vi "PQfetchTables.vi"(8 "error in":errorcluster, 10 "res":u32, 11 "conn":u32) -> (0 "error out":errorcluster, 1 "Data":string[](array[string]), 2 "res_out":u32, 3 "conn_out":u32, 4 "PQnTuples":i32, 6 "PQnFields":i32)   [LabVIEW 2019, in "libpqutility.lvlib"]
doc: "Fetch Result Data from DatabaseRequest into String Array.\nSee PostgreSQL c-lib doku for further information."
uses:
  libpqutility.lvlib
  libpqlv/libpqlv.lvlib
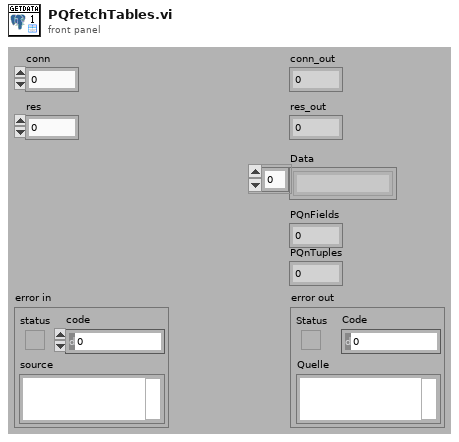
[diagram p1: front panel]
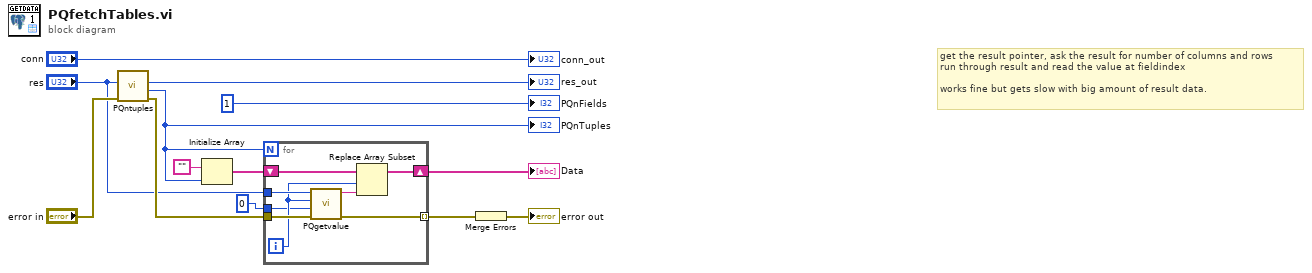
[diagram p0: block diagram]
diagram:
  # "get the result pointer, ask the result for number of columns and rows\nrun through result and read the value at fieldindex\n\nworks fine but gets slow with big amount of result data."
  n1 = call "PQntuples.vi"("error in (no error)"="error in", "res"="res") -> ("error out"=w12:errorcluster, "PQnTuples"=w5:i32, "res out"=→"res_out":u32)  [unwired: 7 in]
  "PQnTuples" <- w5
  n2 = Initialize Array("", w5) -> (w6:string[])
  n3 = for {
    N: w5 -> [_]
    tunnel: "res" -> [w21]
    tunnel: w12 -> [w20]
    tunnel: [w15] -> w4 mode=indexing
    shift-right: [w18] -> w7
    shift-left: w6 -> [w16]
    tunnel: 0 ("column_number") -> [w14]
    i -> [w17]
    n4 = call "PQgetvalue.vi"("error in (no error)"=w20, "column_number"=w14, "row_number"=w17, "res"=w21) -> ("error out"=w15:errorcluster, "field_value"=w19:string)  [unwired: 6 in]
    n5 = Replace Array Subset(array=w16, new element=w19, index=w17) -> (w18:string[])
  }
  "Data" <- w7
  n6 = Merge Errors(w4) -> (→"error out":errorcluster)
  "conn_out" <- "conn"
  "PQnFields" <- 1 ("PQnFields")
